vi "泵温度校准配置.vi"() -> ()   [LabVIEW 2016, in "斯坦道CODMn新电路板.lvlib"]
uses:
  <vilib>/Utility/miscctls.llb/LVPointTypeDef.ctl
panel:
  in  "关闭":bool
  in  "偏心轮校准簇":T1={"复位"=FALSE, "进纯水"=FALSE, "停止"=FALSE, "液体重量"=60, "偏心轮校准"=FALSE}
  in  "温度校准簇":T2={"进纯水"=FALSE, "排液"=FALSE, "停止 2"=FALSE, "开始加热"=FALSE, "温度值"=115.0, "温度校准"=FALSE}
  # "偏心轮、温度校准"
  # "输入实际液体重量:"
  # "g"
  # "温度:"
  # "℃"
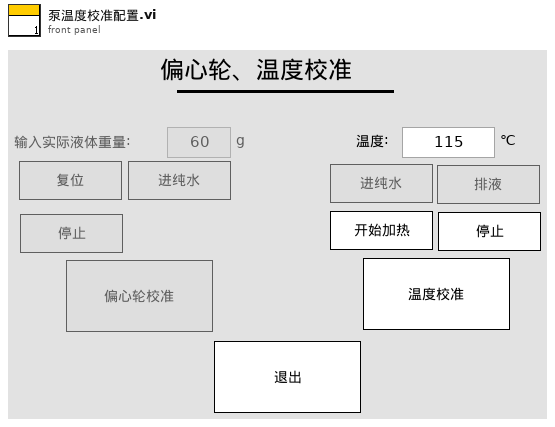
[diagram p1: front panel]
types:
  T1 = cluster{"复位":bool, "进纯水":bool, "停止":bool, "液体重量":u16, "偏心轮校准":bool}
  T2 = cluster{"进纯水":bool, "排液":bool, "停止 2":bool, "开始加热":bool, "温度值":dbl, "温度校准":bool}
  T3 = enum8{"Enabled", "Disabled", "Disabled and Grayed Out"}
  T4 = typedef "LVPointTypeDef.ctl" = cluster{"Horizontal":i16, "Vertical":i16}
  T5 = cluster{"泵类型":u8, "阀数量":u8, "纯水通道":u16, "废液通道":u8, "进样速度":u16, "出样速度":u16, "滴定速度":u16, "注射泵保温温度L":u8, "注射泵保温温度H":u8, "注射泵加热超时时间":u16, "是否存在液位检测板":u16, "A值告警下限值":u16, "A值告警上限值":u16, "B值告警下限值":u16, "B值告警上限值":u16, "AB跨度告警值":u16, "阀配置:":u8, "滴定等待时间":u16, "滴定吸光度斜率":dbl, "传感器阈值":u16}
  T6 = cluster{"系统时间":timestamp, "工作状态":u16, "测量模式":enum16{"待机", "连续模式", "周期模式", "定点模式", "受控模式", "手动模式"}, "告警代码":u16, "故障代码":u16, "日志代码":u16, "软件版本":u16, "A":sgl, "B":sgl, "K":sgl, "当前滴定数":sgl, "T":sgl, "H":sgl, "id":u16, "flowid":u16, "量程":u16, "加热实时温度":sgl, "当前ORP值":sgl, "运行时间":sgl, "当前步骤剩余时间":sgl, "结束滴定数":sgl, "注射泵保温温度":sgl, "匹配滴定数X0":u16, "X^2":sgl, "X":sgl, "B 2":sgl, "光值1":sgl, "光值2":sgl, "光值3":sgl, "光值4":sgl, "光值5":sgl, "光值6":sgl, "光值7":sgl, "光值8":sgl}
  T7 = cluster{"偏心轮校准参数":dbl, "运行速度(修改需要重启)":u16, "加热温度(校准参数) ":dbl, "告警温度":dbl, "加热超时时间:(单位/秒)":dbl, "K p":dbl, "K i":dbl, "K d":dbl, "ILimitUp":dbl, "ILimitDown":dbl}
  T8 = cluster{"检出限":dbl, "测量精度":dbl, "上限":dbl, "下限":dbl, "阈值（低->高）":dbl, "阈值（高->低）":dbl}
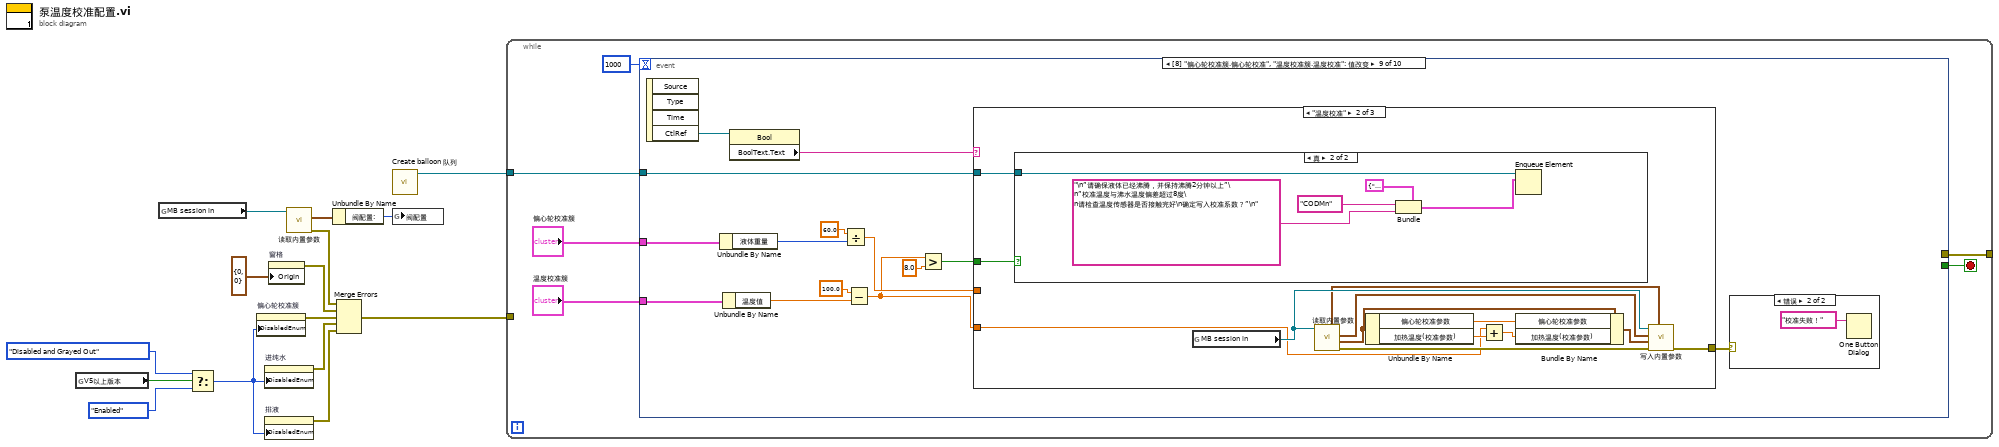
[diagram p0: block diagram]
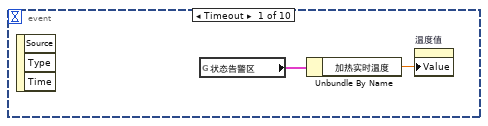
[diagram p2: hidden frame]
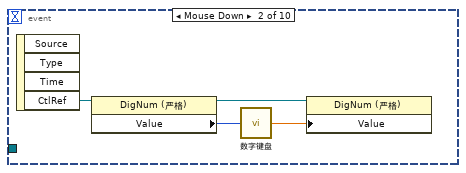
[diagram p3: hidden frame]
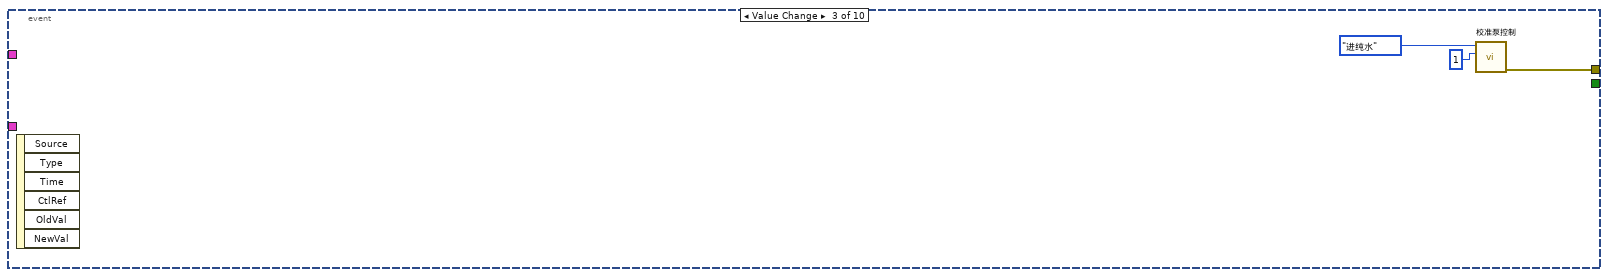
[diagram p4: hidden frame]
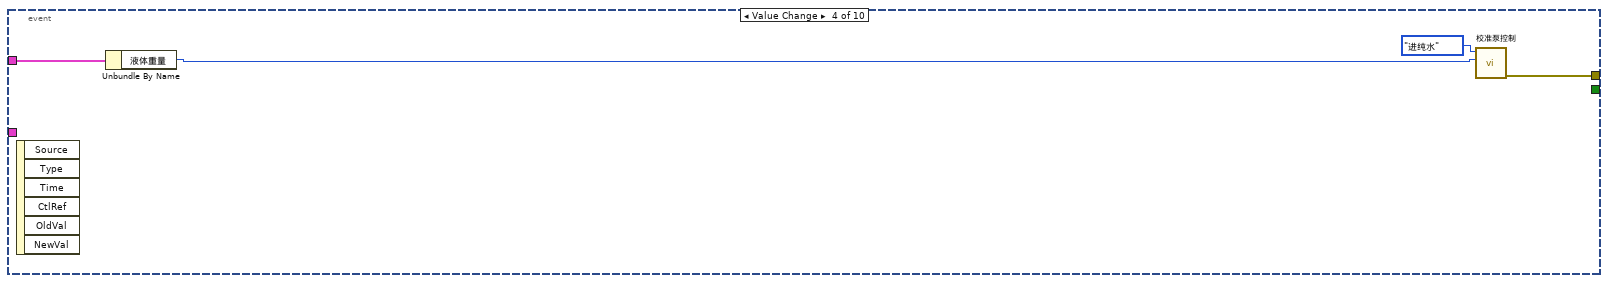
[diagram p5: hidden frame]
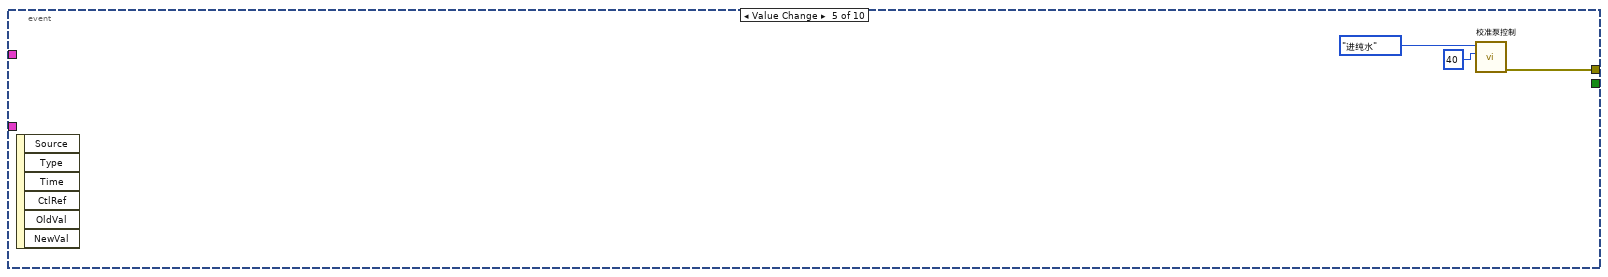
[diagram p6: hidden frame]
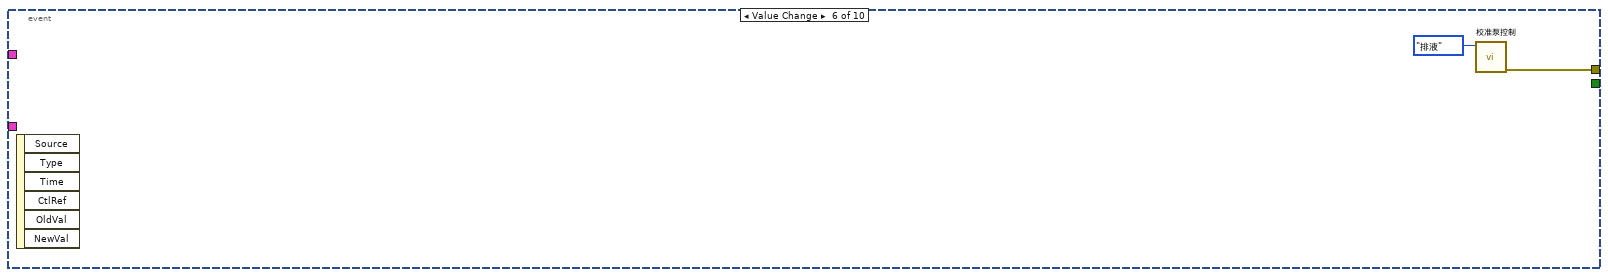
[diagram p7: hidden frame]
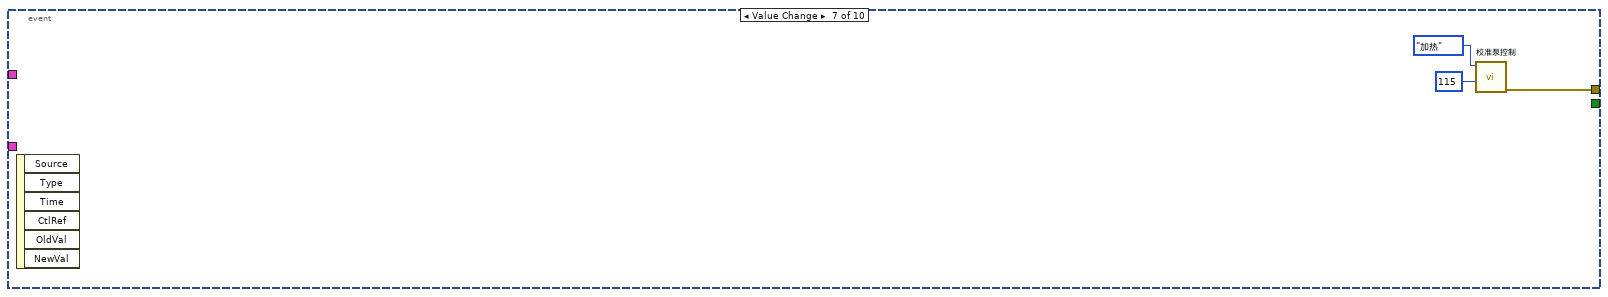
[diagram p8: hidden frame]
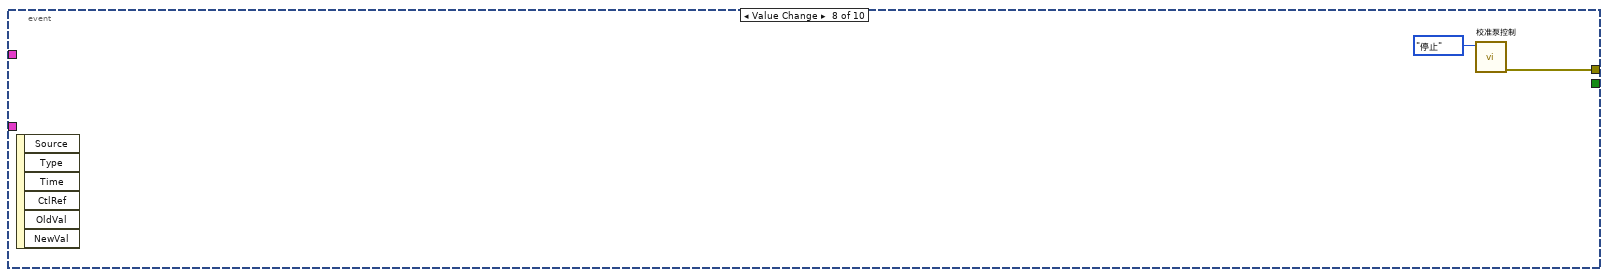
[diagram p9: hidden frame]
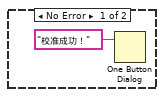
[diagram p10: hidden frame]
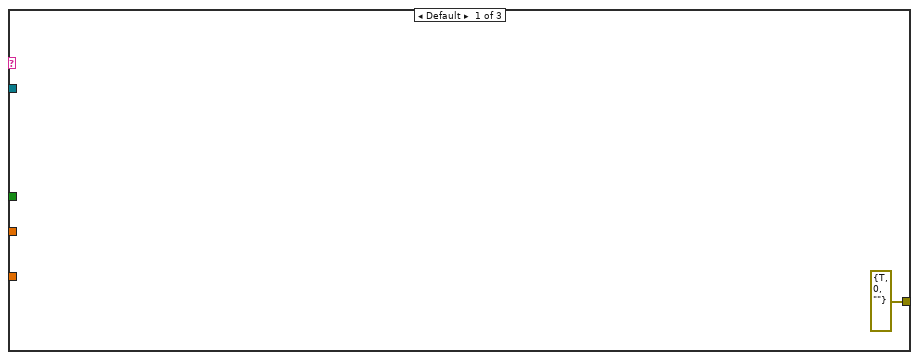
[diagram p11: hidden frame]
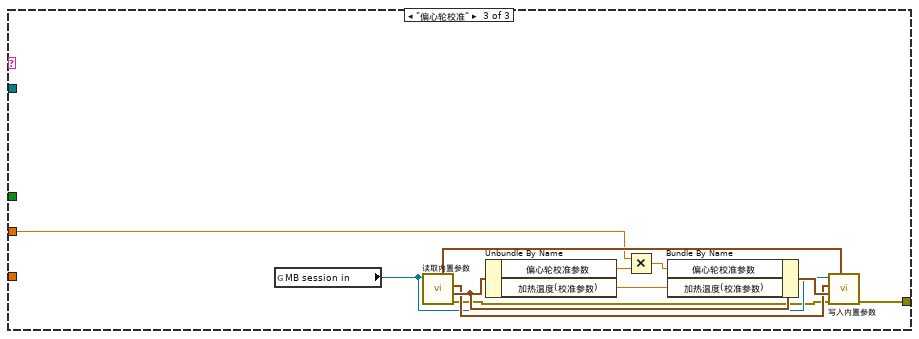
[diagram p13: hidden frame]
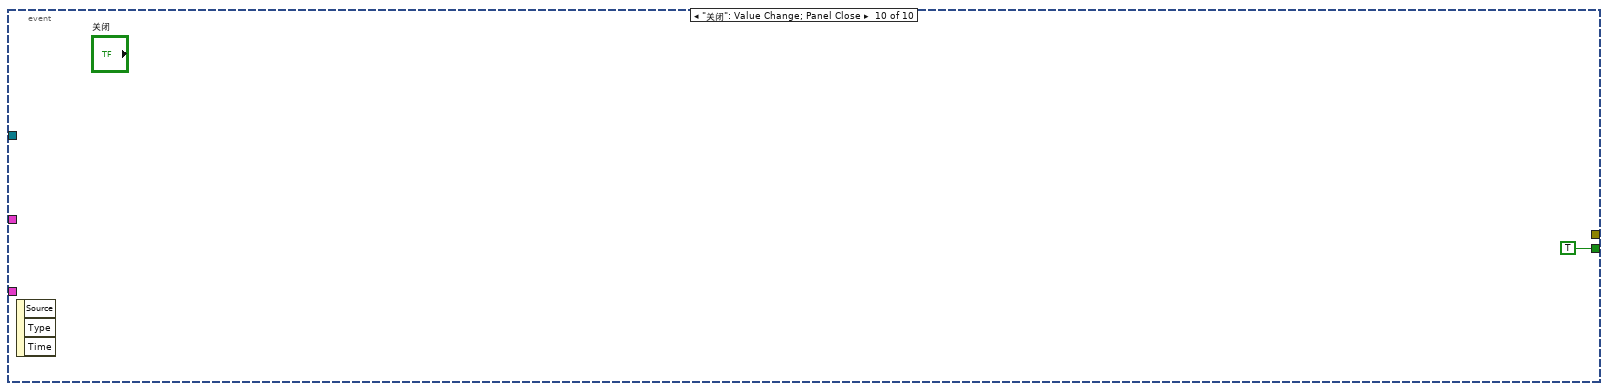
[diagram p14: hidden frame]
diagram:
  n1 = global read "VARCODMn全局变量.vi" "V5以上版本"() -> (w1:bool)
  n2 = global read "VARCODMn全局变量.vi" "MB session in"() -> (w13:refnum<class "MB_Master.lvclass">)
  n3 = Select(t=T3."Disabled and Grayed Out" ("禁用"), s=w1, f=T3."Enabled" ("禁用")) -> (s? t:f=w8:T3)
  n4 = property on="偏心轮校准簇" class="Clust"("DisabledEnum"=w8) -> (error out=w5:errorcluster)  [unwired: 2 in, 1 out]
  n5 = property on="进纯水" class="Bool"("DisabledEnum"=w8) -> (error out=w4:errorcluster)  [unwired: 2 in, 1 out]
  n6 = property on="排液" class="Bool"("DisabledEnum"=w8) -> (error out=w3:errorcluster)  [unwired: 2 in, 1 out]
  n7 = property on="窗格" class="Pane"("Origin"=T4 {"Horizontal"=0, "Vertical"=0} ("原点")) -> (error out=w6:errorcluster)  [unwired: 2 in, 1 out]
  n8 = call "读取内置参数.vi"("MB session in"=w13) -> ("error out"=w7:errorcluster, "外设配置"=w12:T5)  [unwired: 6 in, 3 out]
  n9 = Unbundle By Name(w12) -> ("阀配置:"=w11:u8)
  n10 = Merge Errors(w7, w6, w5, w4, w3) -> (w2:errorcluster)
  n11 = call "Create balloon 队列.vi"() -> ("队列输出"=w14:refnum<queue>)  [unwired: 11 in]
  n12 = global write "CODMn断电保存全局变量.vi" "阀配置"(w11) -> ()
  n13 = while {
    tunnel: [w20] -> _
    tunnel: w14 -> [w18]
    tunnel: w2 -> [_]
    stop <- w21 stop-if-true
    n14 = event shown="[8] \"偏心轮校准簇.偏心轮校准\", \"温度校准簇.温度校准\": 值改变" {
      selector: _ -> [_ _ _ _ _ _ _ _ _ _]
      dyn-events: _ -> [_ _ _ _ _ _ _ _ _ _]
      timeout: 1000 -> [_ _ _ _ _ _ _ _ _ _]
      tunnel: [_ _ _ _ _ _ _ _ _ TRUE] -> w21
      tunnel: "偏心轮校准簇" -> [_ _ _ w33 _ _ _ _ w58 _]
      tunnel: [_ _ w29 w34 w37 w39 w42 w44 _ _] -> w20
      tunnel: "温度校准簇" -> [_ _ _ _ _ _ _ _ w45 _]
      tunnel: w18 -> [_ _ _ _ _ _ _ _ w47 _]
      event Timeout {
        n15 = event-data() -> ()  [unwired: 1 in, 3 out]
        n16 = global read "VARCODMn全局变量.vi" "状态告警区"() -> (w23:T6)
        n17 = Unbundle By Name(w23) -> ("加热实时温度"=w22:sgl)
        n18 = property on="温度值" class="DigNum (严格)"("Value"=w22) -> ()  [unwired: 2 in, 2 out]
      }
      event "偏心轮校准簇.液体重量": Mouse Down {
        n19 = event-data() -> ("CtlRef"=w24:refnum<vi>)  [unwired: 1 in, 3 out]
        n20 = property class="DigNum (严格)"(reference=w24) -> (reference out=w26:refnum<vi>, "Value"=w27:u16)  [unwired: 1 in, 1 out]
        n21 = call "数字键盘.vi"("OldNumber"=w27) -> ("NewNumber"=w25:dbl)
        n22 = property class="DigNum (严格)"(reference=w26, "Value"=w25) -> ()  [unwired: 1 in, 2 out]
      }
      event "偏心轮校准簇.复位": Value Change {
        n23 = event-data() -> ()  [unwired: 1 in, 6 out]
        n24 = call "校准泵控制.vi"("偏心轮"=u16 1, "枚举"=enum16{"进水样", "进纯水", "排液", "加热", "停止"}."进纯水") -> ("错误输出"=w29:errorcluster)  [unwired: 9 in]
      }
      event "偏心轮校准簇.进纯水": Value Change {
        n25 = event-data() -> ()  [unwired: 1 in, 6 out]
        n26 = Unbundle By Name(w33) -> ("液体重量"=w32:u16)
        n27 = call "校准泵控制.vi"("偏心轮"=w32, "枚举"=enum16{"进水样", "进纯水", "排液", "加热", "停止"}."进纯水") -> ("错误输出"=w34:errorcluster)  [unwired: 9 in]
      }
      event "温度校准簇.进纯水": Value Change {
        n28 = event-data() -> ()  [unwired: 1 in, 6 out]
        n29 = call "校准泵控制.vi"("偏心轮"=u16 40, "枚举"=enum16{"进水样", "进纯水", "排液", "加热", "停止"}."进纯水") -> ("错误输出"=w37:errorcluster)  [unwired: 9 in]
      }
      event "温度校准簇.排液": Value Change {
        n30 = event-data() -> ()  [unwired: 1 in, 6 out]
        n31 = call "校准泵控制.vi"("枚举"=enum16{"进水样", "进纯水", "排液", "加热", "停止"}."排液") -> ("错误输出"=w39:errorcluster)  [unwired: 10 in]
      }
      event "温度校准簇.开始加热": Value Change {
        n32 = event-data() -> ()  [unwired: 1 in, 6 out]
        n33 = call "校准泵控制.vi"("摄氏度"=u16 115, "枚举"=enum16{"进水样", "进纯水", "排液", "加热", "停止"}."加热") -> ("错误输出"=w42:errorcluster)  [unwired: 9 in]
      }
      event "温度校准簇.停止 2", "偏心轮校准簇.停止": Value Change {
        n34 = event-data() -> ()  [unwired: 1 in, 6 out]
        n35 = call "校准泵控制.vi"("枚举"=enum16{"进水样", "进纯水", "排液", "加热", "停止"}."停止") -> ("错误输出"=w44:errorcluster)  [unwired: 10 in]
      }
      event "偏心轮校准簇.偏心轮校准", "温度校准簇.温度校准": Value Change {
        n36 = event-data() -> ("CtlRef"=w52:refnum<vi>)  [unwired: 1 in, 3 out]
        n37 = Unbundle By Name(w58) -> ("液体重量"=w56:u16)
        n38 = Unbundle By Name(w45) -> ("温度值"=w54:dbl)
        n39 = property class="Bool"(reference=w52) -> ("BoolText.Text"=w49:string)  [unwired: 1 in, 2 out]
        n40 = Divide(x=60.0, y=w56) -> (x/y=w51:dbl)
        n41 = Subtract(x=100.0, y=w54) -> (x-y=w50:dbl)
        n42 = Greater?(x=w50, y=8.0) -> (0:w48:bool)
        n43 = case shown="\"温度校准\"" w49 {
          tunnel: w51 -> [_ _ w82]
          tunnel: w50 -> [_ w64 _]
          tunnel: w48 -> [_ w66 _]
          tunnel: w47 -> [_ w65 _]
          tunnel: [errorcluster {"status"=TRUE, "code"=0, "source"=""} ("error out") w62 w80] -> w46
          frame Default {
          }
          frame "温度校准" {
            n44 = case shown="真" w66 {
              tunnel: w65 -> [_ w79]
              frame False {
              }
              frame True {
                n45 = Bundle(cluster=cluster{"Title":string, "Body":string} {"Title"="", "Body"=""} ("元素"), "Title"="CODMn", "Body"="\n”请确保液体已经沸腾，并保持沸腾2分钟以上”\n”校准温度与沸水温度偏差超过8度\n请检查温度传感器是否接触完好\n确定写入校准系数？”\n") -> (w75:cluster{"Title":string, "Body":string})
                n46 = Enqueue Element(queue=w79, element=w75) -> ()  [unwired: 2 in, 3 out]
              }
            }
            n47 = global read "VARCODMn全局变量.vi" "MB session in"() -> (w69:refnum<class "MB_Master.lvclass">)
            n48 = call "读取内置参数.vi"("MB session in"=w69) -> ("error out"=w67:errorcluster, "float"=w71:T7, "外设配置"=w70:T5, "量程参数读取"=w68:T8)  [unwired: 6 in, 1 out]
            n49 = Unbundle By Name(w71) -> ("偏心轮校准参数"=w63:dbl, "加热温度(校准参数)"=w73:dbl)
            n50 = Add(x=w64, y=w73) -> (x+y=w74:dbl)
            n51 = Bundle By Name(cluster=w71, "偏心轮校准参数"=w63, "加热温度(校准参数)"=w74) -> (w72:T7)
            n52 = call "写入内置参数.vi"("量程参数读取"=w68, "error in (no error)"=w67, "float"=w72, "外设配置"=w70, "MB session in"=w69) -> ("error out"=w62:errorcluster)  [unwired: 5 in, 1 out]
          }
          frame "偏心轮校准" {
            n53 = global read "VARCODMn全局变量.vi" "MB session in"() -> (w85:refnum<class "MB_Master.lvclass">)
            n54 = call "读取内置参数.vi"("MB session in"=w85) -> ("error out"=w83:errorcluster, "float"=w87:T7, "外设配置"=w86:T5, "量程参数读取"=w84:T8)  [unwired: 6 in, 1 out]
            n55 = Unbundle By Name(w87) -> ("偏心轮校准参数"=w89:dbl, "加热温度(校准参数)"=w81:dbl)
            n56 = Multiply(x=w82, y=w89) -> (x*y=w90:dbl)
            n57 = Bundle By Name(cluster=w87, "偏心轮校准参数"=w90, "加热温度(校准参数)"=w81) -> (w88:T7)
            n58 = call "写入内置参数.vi"("量程参数读取"=w84, "error in (no error)"=w83, "float"=w88, "外设配置"=w86, "MB session in"=w85) -> ("error out"=w80:errorcluster)  [unwired: 5 in, 1 out]
          }
        }
        n59 = case shown="错误" w46 {
          frame No Error {
            n60 = One Button Dialog(message="校准成功！" ("消息")) -> ()  [unwired: 1 in, 1 out]
          }
          frame Error {
            n61 = One Button Dialog(message="校准失败！" ("消息")) -> ()  [unwired: 1 in, 1 out]
          }
        }
      }
      event "关闭": Value Change; Panel Close {
        n62 = event-data() -> ()  [unwired: 1 in, 3 out]
      }
    }
  }
